vi "Actor Core.vi"(8 "error in":errorcluster, 11 "Task in":refnum<class "Task.lvclass">) -> (0 "error out":errorcluster, 3 "Actor out":refnum<class "Actor.lvclass">)   [LabVIEW 2020, in "Volatus.lvlib" / "Task.lvclass"]
doc: "(<B>Filename</B>: Actor Framework.lvlib:Actor.lvclass:Actor Core.vi)\n\nReceives messages to the actor, reacts to them, and initiates any error handling that may shut the actor down.\n\nDescendant classes may override this VI to append parallel tasks for the actor to complete while it handles messages. Overrides use the Call Parent Class Method node."
uses:
  Task.lvclass
  C:/Program Files (x86)/National Instruments/LabVIEW 2020/vi.lib/ActorFramework/Actor/Actor.lvclass
  <vilib>/ActorFramework/Actor/Actor.lvclass
  Task State.ctl
  Event Level.ctl
  Task.lvclass/Task.ctl
  VolatusAPI/VolatusAPI.lvclass/VolatusAPI.ctl
  Event API/EventAPI.lvclass/EventAPI.ctl
  EventHandler Messages/Handle Event Msg/Handle Event Msg.lvclass/Handle Event Msg.ctl
  <vilib>/ActorFramework/Message Enqueuer/Message Enqueuer.lvclass/Message Enqueuer.ctl
  EventHandler Messages/Handle Event Msg/Send Handle Event.vi
  <vilib>/ActorFramework/Message Enqueuer/Enqueue.vi
  EventHandler Messages/Handle Event Msg/Handle Event Msg.lvclass
  C:/Program Files (x86)/National Instruments/LabVIEW 2020/vi.lib/ActorFramework/Message/Message.lvclass
  <vilib>/ActorFramework/Message Priority Queue/Priority Enqueue.vi
  Volatus.lvlib
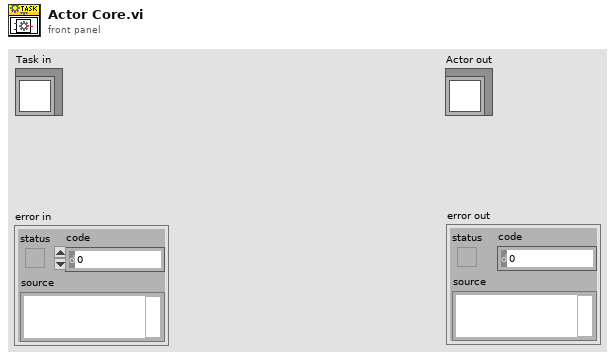
[diagram p1: front panel]
types:
  T1 = typedef "Volatus.lvlib/Event Level.ctl" = enum16{"Debug", "Info", "Warning", "Error"}
  T2 = typedef "Volatus.lvlib/Task State.ctl" = enum16{"Unknown", "Idle", "Initializing", "Starting", "Running", "Stopping", "Stopped", "Error - Init", "Error - Start", "Error - Run", "Error - Stop"}
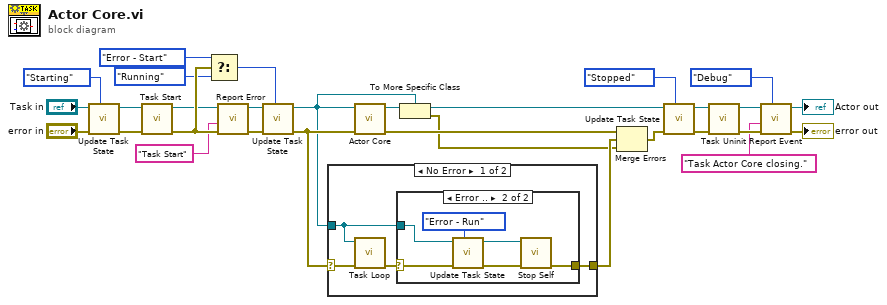
[diagram p0: block diagram]
diagram:
  n1 = call "Update Task State.vi"("State"=Task_State."Starting", "error in (no error)"="error in", "Task in"="Task in") -> ("error out"=w27:errorcluster, "Task out"=w24:refnum<class "Task.lvclass">)  [unwired: 7 in]
  n2 = call-dynamic "Task Start.vi"("error in (no error)"=w27, "Task in"=w24) -> ("error out"=w30:errorcluster, "Task out"=w8:refnum<class "Task.lvclass">)  [unwired: 8 in]
  n3 = Select(t=Task_State."Error - Start", s=w30, f=Task_State."Running" ("State")) -> (s? t:f=w21:T2)
  n4 = call "Report Error.vi"("error in (no error)"=w30, "Message"="Task Start", "Task in"=w8) -> ("error out"=w9:errorcluster, "Task out"=w7:refnum<class "Task.lvclass">)  [unwired: 7 in]
  n5 = call "Update Task State.vi"("State"=w21, "error in (no error)"=w9, "Task in"=w7) -> ("error out"=w20:errorcluster, "Task out"=w14:refnum<class "Task.lvclass">)  [unwired: 7 in]
  n6 = case shown="No Error" w20 {
    selector: w20 -> [w34 _]
    tunnel: w14 -> [w32 _]
    tunnel: [w31 _] -> w18
    frame No Error {
      n7 = call-dynamic "Task Loop.vi"("error in (no error)"=w34, "Task in"=w32) -> ("error out"=w33:errorcluster)  [unwired: 9 in]
      n8 = case shown="Error .." w33 {
        selector: w33 -> [w35 w41]
        tunnel: w32 -> [_ w39]
        tunnel: [w35 w36] -> w31
        frame No Error {
        }
        frame Error {
          n9 = call "Update Task State.vi"("State"=Task_State."Error - Run", "error in (no error)"=w41, "Task in"=w39) -> ("error out"=w37:errorcluster, "Task out"=w38:refnum<class "Task.lvclass">)  [unwired: 7 in]
          n10 = call "Stop Self.vi"("error in (no error)"=w37, "Task in"=w38) -> ("error out"=w36:errorcluster)  [unwired: 8 in, 1 out]
        }
      }
    }
    frame Error {
      # "Don't pass error here, gets forwarded through MHL"
    }
  }
  n11 = call-parent "Actor Core.vi"("error in"=w20, "Actor in"=w14) -> ("error out"=w28:errorcluster, "Actor out"=w16:refnum<class "Actor.lvclass">)  [unwired: 8 in]
  n12 = To More Specific Class(target class=w14, reference=w16) -> (specific class reference=w15:refnum<class "Task.lvclass">, error out=w13:errorcluster)  [unwired: 1 in]
  n13 = Merge Errors(w28, w18, w13) -> (w19:errorcluster)
  n14 = call "Update Task State.vi"("State"=Task_State."Stopped", "error in (no error)"=w19, "Task in"=w15) -> ("error out"=w17:errorcluster, "Task out"=w10:refnum<class "Task.lvclass">)  [unwired: 7 in]
  n15 = call-dynamic "Task Uninit.vi"("error in (no error)"=w17, "Task in"=w10) -> ("error out"=w11:errorcluster, "Task out"=w4:refnum<class "Task.lvclass">)  [unwired: 8 in]
  n16 = call "Report Event.vi"("Level (Info)"=Event_Level."Debug", "error in (no error)"=w11, "Message"="Task Actor Core closing.", "Task in"=w4) -> ("error out"=→"error out":errorcluster, "Task out"=→"Actor out":refnum<class "Task.lvclass">)  [unwired: 6 in]
